vi "Discover Remote Packages.vi"(8 "error in (no error)":errorcluster, 11 "Artifactory.VIPM in":refnum<class "Artifactory.VIPM.lvclass">) -> (0 "error out":errorcluster, 2 "Remote Packages":map{string, string[]}(c390), 3 "Artifactory.VIPM out":refnum<class "Artifactory.VIPM.lvclass">)   [LabVIEW 2021, in "Artifactory.VIPM.lvclass"]
uses:
  Artifactory.VIPM.lvclass
  Artifactory.VIPM.lvclass/Artifactory.VIPM.ctl
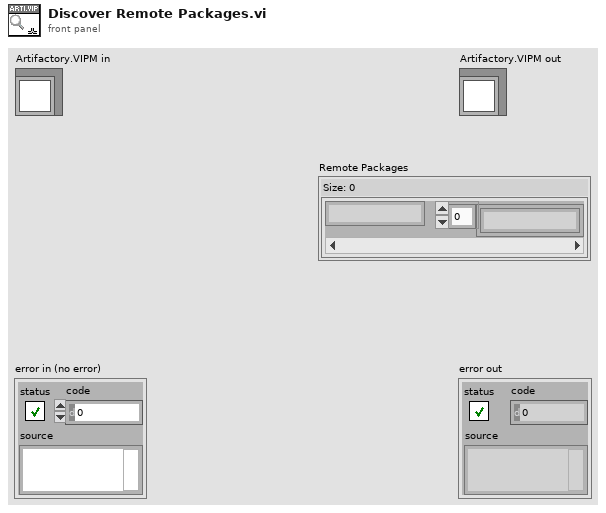
[diagram p1: front panel]
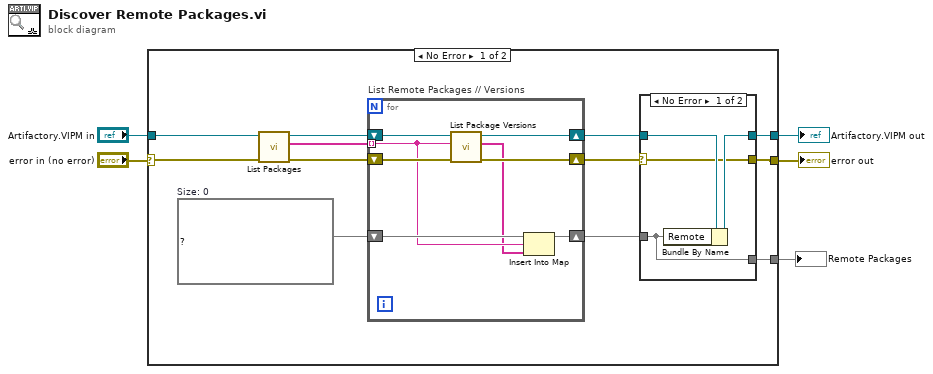
[diagram p0: block diagram]
diagram:
  n1 = case shown="No Error" "error in (no error)" {
    selector: "error in (no error)" -> [w12 w33]
    tunnel: [w8 w33] -> w4
    tunnel: [w9 w32] -> w2
    tunnel: "Artifactory.VIPM in" -> [w13 w32]
    tunnel: [w6 _] -> w1
    frame No Error {
      w14 = map{string, string[]} {}  # Size: 0
      n2 = call "List Packages.vi"("error in (no error)"=w12, "Artifactory.VIPM in"=w13) -> ("error out"=w16:errorcluster, "VI Packages"=w15:string[], "Artifactory.VIPM out"=w17:refnum<class "Artifactory.VIPM.lvclass">)  [unwired: 6 in, 1 out]
      n3 = for "List Remote Packages // Versions" {
        shift-right: [w30] -> w10
        shift-left: w17 -> [w31]
        tunnel: w15 -> [w26] mode=indexing
        shift-right: [w24] -> w11
        shift-left: w14 -> [w27]
        shift-right: [w28] -> w7
        shift-left: w16 -> [w29]
        n4 = call "List Package Versions.vi"("error in (no error)"=w29, "Package Name"=w26, "Artifactory.VIPM in"=w31) -> ("error out"=w28:errorcluster, "Package Versions"=w25:string[], "Artifactory.VIPM out"=w30:refnum<class "Artifactory.VIPM.lvclass">)  [unwired: 5 in, 1 out]
        n5 = Insert Into Map(map in=w27, key=w26, value=w25) -> (map out=w24:map{string, string[]})  [unwired: 2 out]
      }
      n6 = case shown="No Error" w7 {
        selector: w7 -> [w19 w22]
        tunnel: w11 -> [w18 _]
        tunnel: w10 -> [w21 w23]
        tunnel: [w20 w23] -> w9
        tunnel: [w19 w22] -> w8
        tunnel: [w18 _] -> w6
        frame No Error {
          n7 = Bundle By Name(cluster=w21, "Remote"=w18) -> (w20:refnum<class "Artifactory.VIPM.lvclass">)
        }
        frame Error {
        }
      }
    }
    frame Error {
    }
  }
  "error out" <- w4
  "Artifactory.VIPM out" <- w2
  "Remote Packages" <- w1
